vi "FGV.vi"(8 "error in (no error)":errorcluster, 10 "FGV_State":T1) -> (0 "error out":errorcluster, 3 "FGV 2":T2 {"Database"."Balance" format="%#.2f"; "Database"."Account Number" format="%_1f"})   [LabVIEW 2020]
doc: "FGV is used to manage all data configuration as Events ref , Queue message handling ref and DB (Read / update)"
uses:
  Controls/FGV_Data.ctl
  SubVIs/Message Queue/All Message Queues.ctl
  SubVIs/Message Queue/Message Cluster.ctl
  Controls/Events_User.ctl
  Database/Controls/Account Database.ctl
  Controls/FGV_State.ctl
  Database/Controls/Todo.ctl
  Controls/Data_Initialize.ctl
  SubVIs/User Event - Stop/User Event - Stop.lvlib
  SubVIs/Message Queue/Message Queue.lvlib
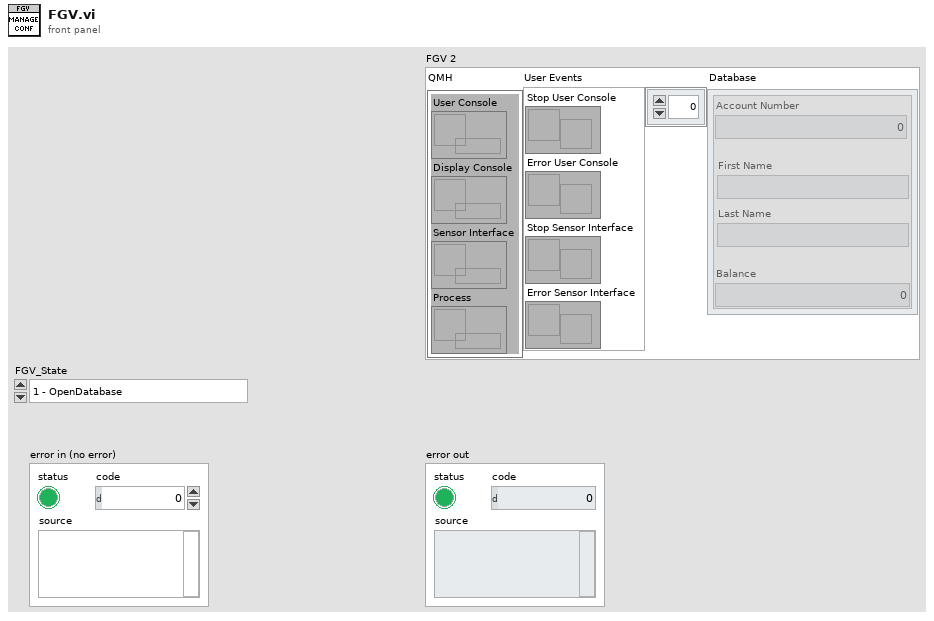
[diagram p1: front panel]
types:
  T1 = typedef "FGV_State.ctl" = enum16{"1 - OpenDatabase", "2 - Initialize Events", "3 - Initialize QMH", "4 - Close QMH", "5 - Close Events", "Read FGV", "Save Database", "Def"}
  T2 = typedef "FGV_Data.ctl" = cluster{"QMH":T3, "User Events":T4, "Database":T5[]}
  T3 = typedef "Message Queue.lvlib/All Message Queues.ctl" = cluster{"User Console":refnum<queue>, "Display Console":refnum<queue>, "Sensor Interface":refnum<queue>, "Process":refnum<queue>}
  T4 = typedef "Events_User.ctl" = cluster{"Stop User Console":refnum<user-event>, "Error User Console":refnum<user-event>, "Stop Sensor Interface ":refnum<user-event>, "Error Sensor Interface":refnum<user-event>}
  T5 = typedef "Account Database.ctl" = cluster{"Account Number":i32, "First Name":string, "Last Name":string, "Balance":dbl}
  T6 = typedef "Todo.ctl" = enum16{"Read", "Update"}
  T7 = typedef "Data_Initialize.ctl" = cluster{"Database":T5[], "User Events":T4}
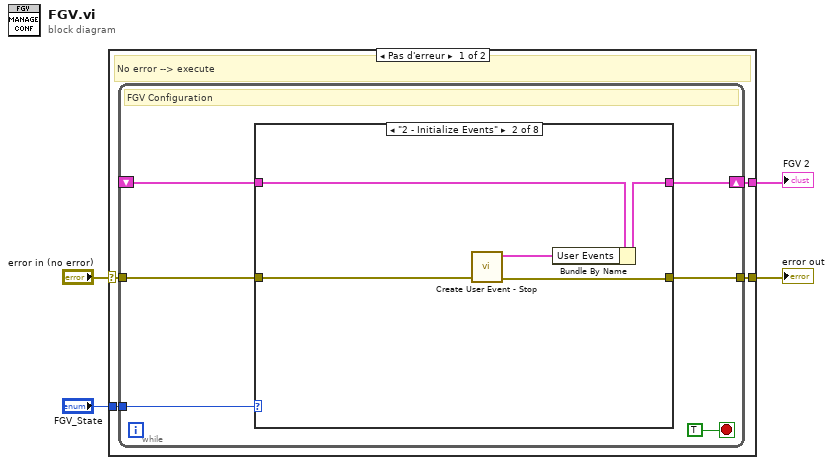
[diagram p0: block diagram]
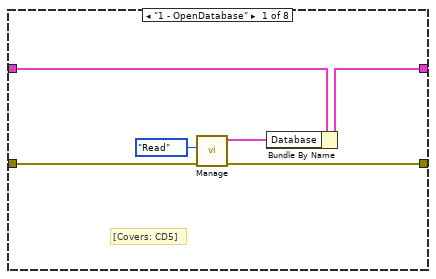
[diagram p2: hidden frame]
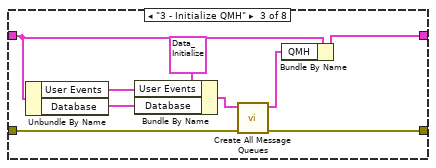
[diagram p3: hidden frame]
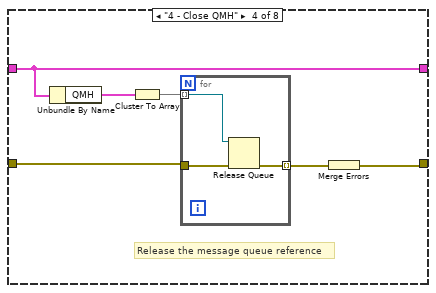
[diagram p4: hidden frame]
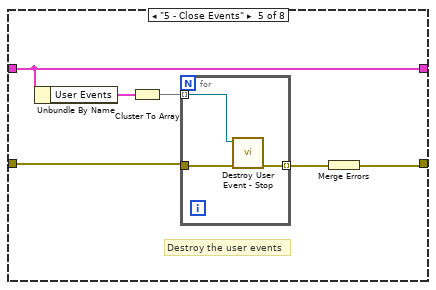
[diagram p5: hidden frame]
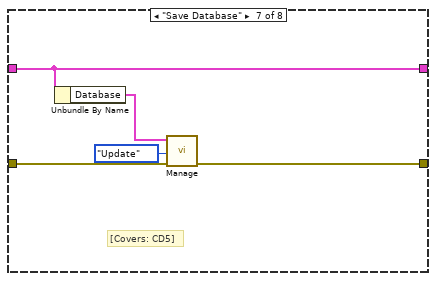
[diagram p7: hidden frame]
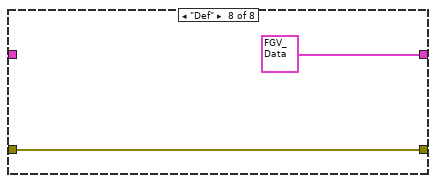
[diagram p8: hidden frame]
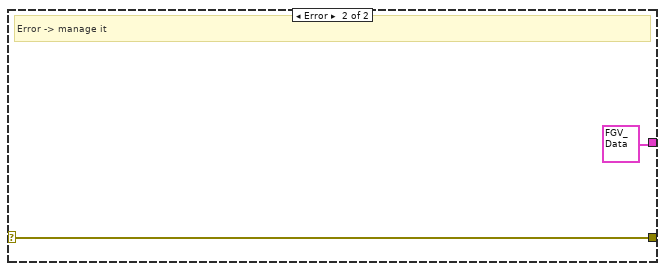
[diagram p9: hidden frame]
diagram:
  n1 = case shown="Pas d'erreur" "error in (no error)" {
    selector: "error in (no error)" -> [w6 w63]
    tunnel: [w8 T2 {"QMH"={"User Console"=refnum, "Display Console"=refnum, "Sensor Interface"=refnum, "Process"=refnum}, "User Events"={"Stop User Console"=refnum, "Error User Console"=refnum, "Stop Sensor Interface "=refnum, "Error Sensor Interface"=refnum}, "Database"=[]} ("FGV 2")] -> w4
    tunnel: [w7 w63] -> w3
    tunnel: "FGV_State" -> [w5 _]
    frame No Error {
      # "No error --> execute"
      n2 = while {
        tunnel: w5 -> [w13]
        shift-right: [w11] -> w8
        shift-left: _ -> [w12]
        tunnel: w6 -> [w10]
        tunnel: [w9] -> w7
        stop <- TRUE stop-if-true
        # "FGV Configuration"
        n3 = case shown="\"2 - Initialize Events\"" w13 {
          tunnel: w12 -> [w20 w23 w28 w39 w48 w54 w59 _]
          tunnel: [w17 w22 w32 w39 w48 w54 w59 T2 {"QMH"={"User Console"=refnum, "Display Console"=refnum, "Sensor Interface"=refnum, "Process"=refnum}, "User Events"={"Stop User Console"=refnum, "Error User Console"=refnum, "Stop Sensor Interface "=refnum, "Error Sensor Interface"=refnum}, "Database"=[]} ("FGV 2")] -> w11
          tunnel: w10 -> [w19 w25 w34 w40 w49 w53 w56 w61]
          tunnel: [w18 w24 w33 w35 w44 w53 w55 w61] -> w9
          frame "1 - OpenDatabase" {
            # "[Covers: CD5]"
            n4 = call "Manage.vi"("error in"=w19, "ToDo"=Todo."Read") -> ("error out"=w18:errorcluster, "Database OUT"=w16:T5[])  [unwired: 8 in]
            n5 = Bundle By Name(cluster=w20, "Database"=w16) -> (w17:T2)
          }
          frame "2 - Initialize Events" {
            n6 = call "Create User Event - Stop.vi"("error in (no error)"=w25) -> ("error out"=w24:errorcluster, "User Events"=w21:T4)  [unwired: 9 in]
            n7 = Bundle By Name(cluster=w23, "User Events"=w21) -> (w22:T2)
          }
          frame "3 - Initialize QMH" {
            n8 = Unbundle By Name(w28) -> ("User Events"=w26:T4, "Database"=w27:T5[])
            n9 = Bundle By Name(cluster=T7 {"Database"=[], "User Events"={"Stop User Console"=refnum, "Error User Console"=refnum, "Stop Sensor Interface "=refnum, "Error Sensor Interface"=refnum}} ("Initiliaze"), "User Events"=w26, "Database"=w27) -> (w29:T7)
            n10 = call "Create All Message Queues.vi"("error in (no error)"=w34, "Initiliaze"=w29) -> ("error out"=w33:errorcluster, "QMH"=w31:T3)  [unwired: 8 in]
            n11 = Bundle By Name(cluster=w28, "QMH"=w31) -> (w32:T2)
          }
          frame "4 - Close QMH" {
            # "Release the message queue reference"
            n12 = Unbundle By Name(w39) -> ("QMH"=w38:T3)
            n13 = Cluster To Array(cluster=w38) -> (array=w37:refnum<queue>[])
            n14 = for {
              tunnel: w37 -> [w41] mode=indexing
              tunnel: w40 -> [w43]
              tunnel: [w42] -> w36 mode=indexing
              n15 = Release Queue(queue=w41, error in (no error)=w43) -> (error out=w42:errorcluster)  [unwired: 1 in, 2 out]
            }
            n16 = Merge Errors(w36) -> (w35:errorcluster)
          }
          frame "5 - Close Events" {
            # "Destroy the user events"
            n17 = Unbundle By Name(w48) -> ("User Events"=w47:T4)
            n18 = Cluster To Array(cluster=w47) -> (array=w46:refnum<user-event>[])
            n19 = for {
              tunnel: w46 -> [w52] mode=indexing
              tunnel: w49 -> [w51]
              tunnel: [w50] -> w45 mode=indexing
              n20 = call "Destroy User Event - Stop.vi"("error in (no error)"=w51, "User Event - Stop"=w52) -> ("error out"=w50:errorcluster)  [unwired: 9 in]
            }
            n21 = Merge Errors(w45) -> (w44:errorcluster)
          }
          frame "Read FGV", Default {
          }
          frame "Save Database" {
            # "[Covers: CD5]"
            n22 = Unbundle By Name(w59) -> ("Database"=w58:T5[])
            n23 = call "Manage.vi"("error in"=w56, "ToDo"=Todo."Update", "Database IN"=w58) -> ("error out"=w55:errorcluster)  [unwired: 7 in, 1 out]
          }
          frame "Def" {
          }
        }
      }
    }
    frame Error {
      # "Error -> manage it"
    }
  }
  "FGV 2" <- w4
  "error out" <- w3
